vi "Execute Acyclic Frame Loopback.vi"(5 "Trigger name":string, 7 "base name for channel aliases":string, 8 "error in":errorcluster, 9 "Rx address base":string, 10 "Tx address base":string, 11 "Loopback in":refnum<class "Loopback.lvclass">) -> (0 "error out":errorcluster, 3 "Loopback out":refnum<class "Loopback.lvclass">)   [LabVIEW 2020, in "Loopback.lvclass"]
uses:
  Loopback.lvclass
  <vilib>/NI/VeriStand Custom Device Testing Tools/VeriStandTestUtilities/VeriStandTestUtilities.lvlib
  <vilib>/NI VeriStand/Execution/Workspace/NI_VS Workspace ExecutionAPI.lvlib
  <vilib>/NI VeriStand/Execution/Workspace/NI VeriStand - Set Single Channel Value.vi
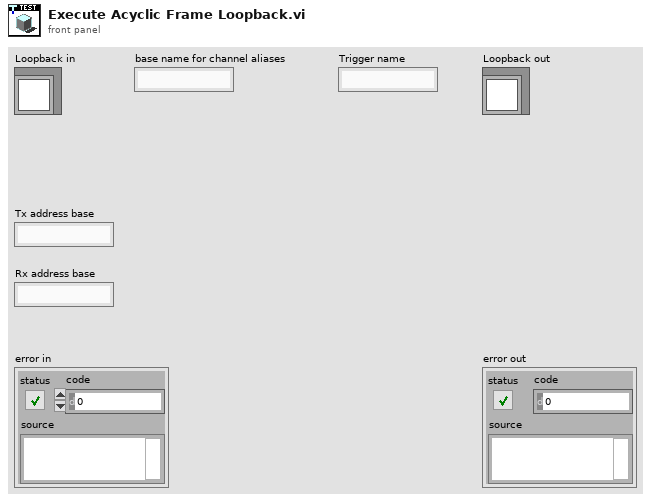
[diagram p1: front panel]
types:
  T1 = typedef "NI_VS Workspace ExecutionAPI.lvlib/WorkspaceAPI.ctl" = refnum<k24>
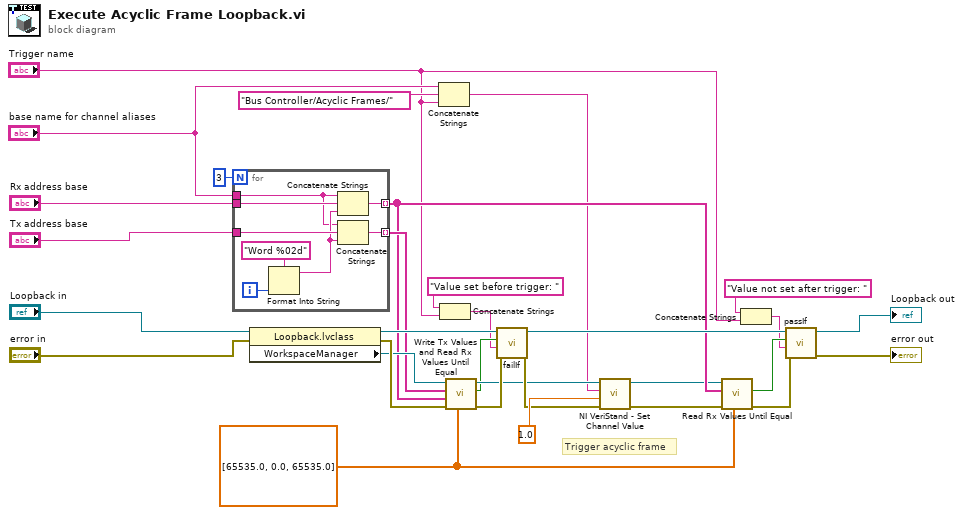
[diagram p0: block diagram]
diagram:
  w11 = dbl[] [65535.0, 0.0, 65535.0]
  # "Trigger acyclic frame"
  n1 = for {
    N: 3 -> [_]
    tunnel: "Tx address base" -> [w38]
    tunnel: [w39] -> w20 mode=indexing
    tunnel: "Rx address base" -> [w37]
    tunnel: [w36] -> w18 mode=indexing
    tunnel: "base name for channel aliases" -> [w32]
    i -> [w35]
    n2 = Format Into String(format string="Word %02d", w35) -> (resulting string=w34:string)  [unwired: 2 in, 1 out]
    n3 = Concatenate Strings(w32, w37, w34) -> (w36:string)
    n4 = Concatenate Strings(w32, w38, w34) -> (w39:string)
  }
  n5 = property class="Loopback.lvclass"(reference="Loopback in", error in="error in") -> (reference out=w31:refnum<class "Loopback.lvclass">, error out=w30:errorcluster, "WorkspaceManager"=w27:T1)
  n6 = Concatenate Strings("base name for channel aliases", "Bus Controller/Acyclic Frames/" ("string"), "Trigger name") -> (w6:string)
  n7 = Concatenate Strings("Value set before trigger: " ("message (\"\")"), "Trigger name") -> (w1:string)
  n8 = call <vilib>:"Write Tx Values and Read Rx Values Until Equal.vi"("Tx values"=w11, "error in"=w30, "Rx aliases"=w18, "Tx aliases"=w20, "workspace manager in"=w27) -> ("error out"=w19:errorcluster, "values equal"=w12:bool, "workspace manager out"=w16:T1)  [unwired: 4 in]
  n9 = call-dynamic "failIf.vi"("error in (no error)"=w19, "message (\"\")"=w1, "fail"=w12, "TestCase in"=w31) -> ("error out"=w22:errorcluster, "TestCase out"=w21:refnum<class "Loopback.lvclass">)  [unwired: 6 in]
  n10 = call-poly <vilib>:"NI VeriStand - Set Channel Value.vi"("error in (no error)"=w22, "Value"=1.0, "Channel"=w6, "WorkspaceManager in"=w16) -> ("error out"=w13:errorcluster, "WorkspaceManager out"=w14:T1)  [unwired: 6 in]
  n11 = call <vilib>:"Read Rx Values Until Equal.vi"("expected values"=w11, "error in"=w13, "Rx aliases"=w18, "workspace manager in"=w14) -> ("error out"=w15:errorcluster, "values equal expected"=w17:bool)  [unwired: 5 in, 1 out]
  n12 = Concatenate Strings("Value not set after trigger: " ("message (\"\")"), "Trigger name") -> (w2:string)
  n13 = call-dynamic "passIf.vi"("error in (no error)"=w15, "message (\"\")"=w2, "pass"=w17, "TestCase in"=w21) -> ("error out"=→"error out":errorcluster, "TestCase out"=→"Loopback out":refnum<class "Loopback.lvclass">)  [unwired: 6 in]
